vi "Nominal to Binary.vi"(0 "Target Type":T1(ring), 5 "Calibration":cluster{"LSB Weight":u32, "Offset":i32}, 9 "Nominal Value":dbl[](array[numeric])) -> (10 "Binary Value":i32[](array[numeric]))   [LabVIEW 2023]
doc: "This VI converts a nominal value to the corresponding binary code."
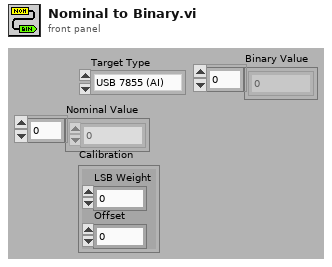
[diagram p1: front panel]
types:
  T1 = enum16{"USB 7855 (AI)", "USB 7855 (AO)", "USB 7855 OEM (AI)", "USB 7855 OEM (AO)", "USB 7856  (AI)", "USB 7856 (AO)", "USB 7856 OEM (AI)", "USB 7856 OEM (AO)"}
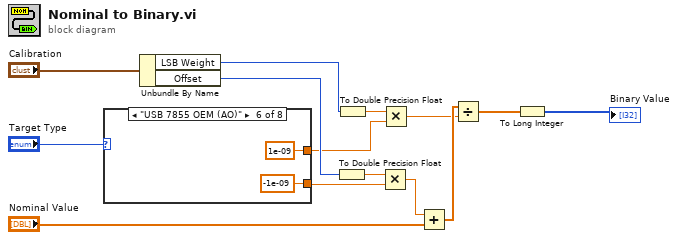
[diagram p0: block diagram]
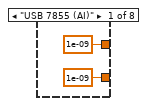
[diagram p2: hidden frame]
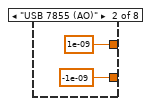
[diagram p3: hidden frame]
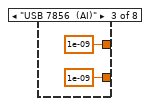
[diagram p4: hidden frame]
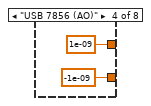
[diagram p5: hidden frame]
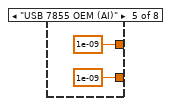
[diagram p6: hidden frame]
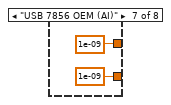
[diagram p7: hidden frame]
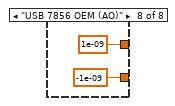
[diagram p8: hidden frame]
diagram:
  n1 = case shown="\"USB 7855 OEM (AO)\"" "Target Type" {
    tunnel: [1e-09 ("y") 1e-09 ("y") 1e-09 ("y") 1e-09 ("y") 1e-09 ("y") 1e-09 ("y") 1e-09 ("y") 1e-09 ("y")] -> w4
    tunnel: [1e-09 ("y") -1e-09 ("y") 1e-09 ("y") -1e-09 ("y") 1e-09 ("y") -1e-09 ("y") 1e-09 ("y") -1e-09 ("y")] -> w3
    frame "USB 7855 (AI)" {
    }
    frame "USB 7855 (AO)" {
    }
    frame "USB 7856  (AI)" {
    }
    frame "USB 7856 (AO)" {
    }
    frame "USB 7855 OEM (AI)" {
    }
    frame "USB 7855 OEM (AO)" {
    }
    frame "USB 7856 OEM (AI)" {
    }
    frame "USB 7856 OEM (AO)" {
    }
  }
  n2 = Unbundle By Name("Calibration") -> ("LSB Weight"=w5:u32, "Offset"=w6:i32)
  n3 = To Double Precision Float(number=w6) -> (double precision float=w9:dbl)
  n4 = To Double Precision Float(number=w5) -> (double precision float=w8:dbl)
  n5 = Multiply(x=w9, y=w3) -> (x*y=w12:dbl)
  n6 = Multiply(x=w8, y=w4) -> (x*y=w13:dbl)
  n7 = Add(x=w12, y="Nominal Value") -> (x+y=w14:dbl[])
  n8 = Divide(x=w14, y=w13) -> (x/y=w2:dbl[])
  n9 = To Long Integer(number=w2) -> (32bit integer=→"Binary Value":i32[])
